vi "Configure Sequencer List All ARB Cycles.vi"(7 "ARB Cycles":i32[](array[numeric]), 8 "error in (no error)":errorcluster, 10 "Instance (1)":i32=1, 11 "VISA resource name":refnum<visa-resource-name>) -> (0 "error out":errorcluster, 3 "VISA resource name out":refnum<visa-resource-name>)   [LabVIEW 2015, in "Rohde&Schwarz CMXP GPRF.lvlib"]
doc: "Defines the ARB cycles for all sequencer list entries.\n\nAttribute:\nRSCMXPGPRF_ATTR_SEQUENCER_LIST_ALL_ARB_CYCLES\n\nRemote-control command:\nSOURce:GPRF:GEN<i>:SEQuencer:LIST:ACYCles:ALL"
uses:
  <instrlib>/Rohde&Schwarz CMXP GPRF/Rohde&Schwarz CMXP GPRF.lvlib
  <instrlib>/Rohde&Schwarz CMXP GPRF/Private/rsidr_core.llb/rsidr_core.lvlib
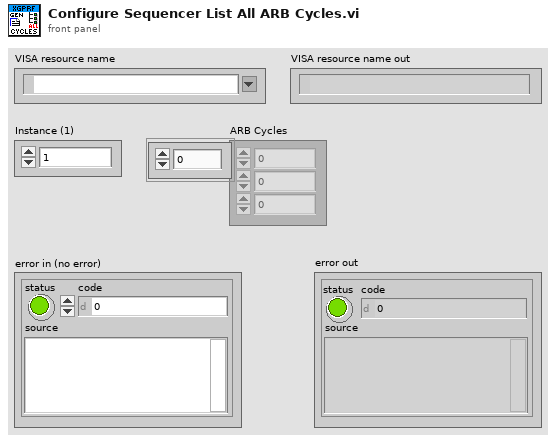
[diagram p1: front panel]
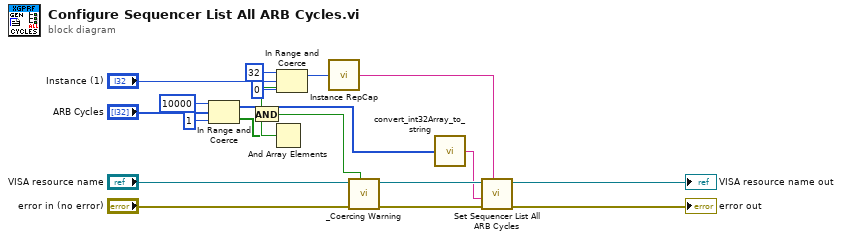
[diagram p0: block diagram]
diagram:
  n1 = In Range and Coerce(upper limit=10000, x="ARB Cycles", lower limit=1) -> (coerced(x)=w11:i32[], In Range?=w8:bool[])
  n2 = And Array Elements(Boolean array=w8) -> (logical AND=w16:bool)
  n3 = In Range and Coerce(upper limit=32, x="Instance (1)", lower limit=0) -> (coerced(x)=w7:i32, In Range?=w18:bool)
  n4 = And(x=w18, y=w16) -> (x .and. y?=w17:bool)
  n5 = call <instrlib>:"Instance RepCap.vi"("instance  in"=w7) -> ("instance out"=w2:string)
  n6 = call <instrlib>:"_Coercing Warning.vi"("In Range?"=w17, "error in (no error)"="error in (no error)", "VISA resource name"="VISA resource name") -> ("error out"=w6:errorcluster, "VISA resource name out"=w5:refnum<visa-resource-name>)  [unwired: 7 in]
  n7 = call <instrlib>:"convert_int32Array_to_string.vi"("I32 array in"=w11) -> ("string out"=w1:string)  [unwired: 4 in]
  n8 = call "Set Sequencer List All ARB Cycles"("Repeated Capabilities"=w2, "error in (no error)"=w6, "Sequencer List All ARB Cycles ()"=w1, "instrument handle"=w5) -> ("error out"=→"error out":errorcluster, "instrument handle out"=→"VISA resource name out":refnum<visa-resource-name>)  [unwired: 6 in]
